vi "Start_Here.vi"() -> ()   [LabVIEW 2019]
panel:
  in  "Open Button":bool
  in  "VI Examples":u16(ring) items=["01 Controls and Indicators.vi", "02 Tools, Colors, and Clicks.vi", "03 Charts.vi", "04 Loops.vi", "05 Graphs.vi", "06 Shift Registers.vi", "07 Arrays.vi", "08 Strings.vi", "09 Clusters.vi", "10 Rings, Strings, and Tables.vi", "11 Execution Order.vi", "12 Events.vi", "13 Case Structures.vi", "14 Saving and Reading Files.vi", "15 Messing with Time.vi", "16 JSON Packets.vi", "21 Talking Serial.vi", "22 RESTful API.vi", "23 Python Node.vi", "24 OS Commands.vi", "51 Simple Queues.vi", "52 Properties.vi", "53 Invoke.vi", "54 Occurences and more.vi", "55 Channels.vi", "56 Panels in panels.vi", "57 Scripting.vi", "71 MP_Reading a voltage.vi", "72 MP_Setting a servo.vi", "81 Arduino_Reading a voltage.vi", "82 Arduino_Setting a servo.vi", "91 WIO_Reading a voltage.vi", "92 WIO_Setting a Servo.vi"]
  # "Getting Started with LabVIEW\n\n1. Select an example\n2. Hit Open and try it out\n3. Close this window when you are done"
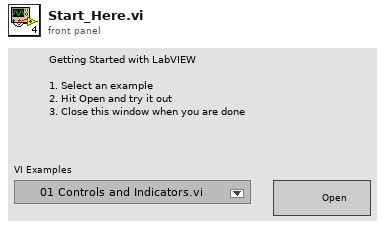
[diagram p1: front panel]
types:
  T1 = enum32{"Invalid", "Standard", "Closed", "Hidden", "Minimized", "Maximized"}
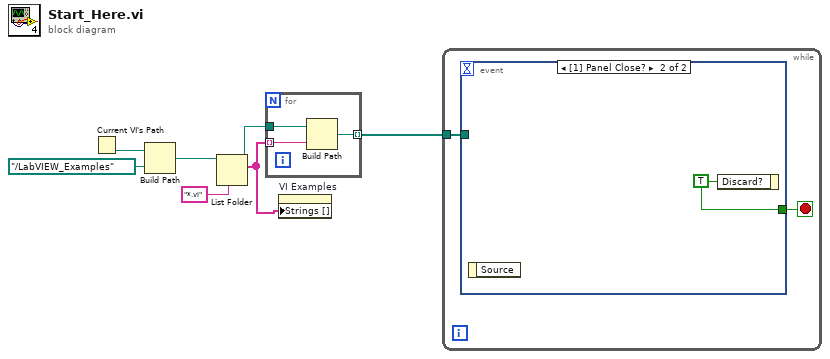
[diagram p0: block diagram]
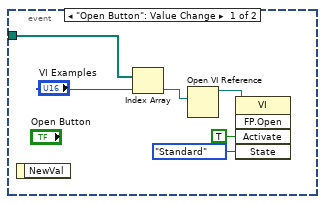
[diagram p2: hidden frame]
diagram:
  n1 = Current VI's Path() -> (path=w4:path)
  n2 = Build Path(base path=w4, name or relative path=path "../LabVIEW_Examples") -> (appended path=w5:path)
  n3 = List Folder(path=w5, pattern="*.vi") -> (path out=w6:path, filenames=w1:string[])  [unwired: 2 in, 2 out]
  n4 = for {
    tunnel: w6 -> [w10]
    tunnel: w1 -> [w9] mode=indexing
    tunnel: [w8] -> w2 mode=indexing
    n5 = Build Path(base path=w10, name or relative path=w9) -> (appended path=w8:path)
  }
  n6 = property on="VI Examples" class="Ring (strict)"("Strings []"=w1) -> ()  [unwired: 2 in, 2 out]
  n7 = while {
    tunnel: w2 -> [w12]
    stop <- w11 stop-if-true
    n8 = event shown="[1] Panel Close?" {
      selector: _ -> [_ _]
      dyn-events: _ -> [_ _]
      timeout: _ -> [_ _]
      tunnel: w12 -> [w13 _]
      tunnel: [_ w19] -> w11
      event "Open Button": Value Change {
        n9 = event-data() -> ()  [unwired: 1 in, 1 out]
        n10 = Index Array(array=w13, index="VI Examples") -> (element=w18:path)
        n11 = Open VI Reference(vi path=w18) -> (vi reference=w16:refnum<vi>)  [unwired: 5 in, 1 out]
        n12 = invoke class="VI" method="FP.Open"(reference=w16, "Activate"=TRUE ("Activate?"), "State"=T1."Standard") -> ()  [unwired: 2 in, 5 out]
      }
      event Panel Close? {
        w19 = TRUE ("Discard?")
        n13 = event-data() -> ()  [unwired: 1 in, 1 out]
        n14 = event-data("Discard?"=w19) -> ()  [unwired: 1 in, 1 out]
      }
    }
  }
